vi "4-3.vi"(1 "字符串":string, 2 "输入":dbl) -> (0 "输出 2":dbl)   [LabVIEW 2017]
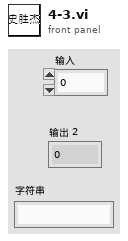
[diagram p1: front panel]
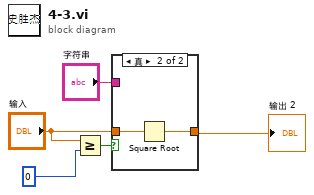
[diagram p0: block diagram]
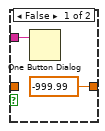
[diagram p2: hidden frame]
diagram:
  n1 = Greater Or Equal?(x="输入", y=0) -> (x >= y?=w4:bool)
  n2 = case shown="真" w4 {
    tunnel: "输入" -> [_ w9]
    tunnel: [-999.99 w8] -> w2
    tunnel: "字符串" -> [w6 _]
    frame False {
      n3 = One Button Dialog(message=w6) -> ()  [unwired: 1 in, 1 out]
    }
    frame True {
      n4 = Square Root(x=w9) -> (sqrt(x)=w8:dbl)
    }
  }
  "输出 2" <- w2
